vi "GF_ConfigTop16fromFile.vi"(11 "Path":path=path "N:/Configuration/Top16Config.csv") -> (2 "Top16 Array":T2(array[cluster]) {"Slope Array" format="%#.6f"; "Dig or An" format="%x"})   [LabVIEW 2016]
uses:
  <vilib>/Utility/file.llb/Read From Spreadsheet File (string).vi
panel:
  in  "Top16Cluster":T1={"Board Name"="FTSK6X4A", "Gain Array"=[0], " Slope Array"=[0.1, 0.2, 0.5, 1.0, 2.0, 5.0, 10.0, 20.0], "Offset Array"=[0.2], "Dig or An"=255, "Handle"=0, "Return"=FALSE}
  out "Rebuilt Array":string[][][](array[string])
  out "Output Array":string[][](array[string])
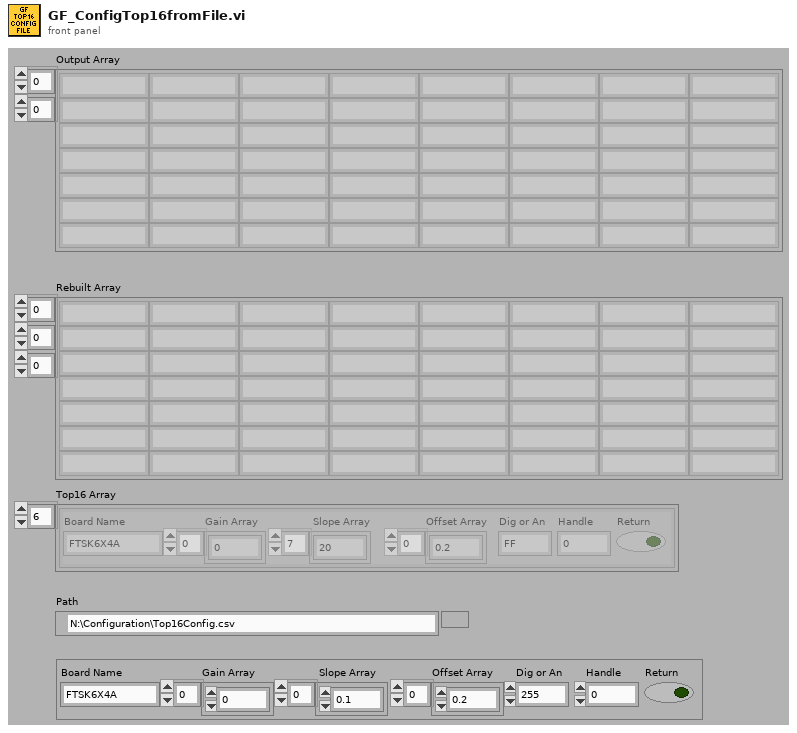
[diagram p1: front panel]
types:
  T1 = cluster{"Board Name":string, "Gain Array":u16[], " Slope Array":dbl[], "Offset Array":dbl[], "Dig or An":u8, "Handle":u32, "Return":bool}
  T2 = cluster{"Board Name":string, "Gain Array":u16[], " Slope Array":dbl[], "Offset Array":dbl[], "Dig or An":u8, "Handle":u32, "Return":bool}[]
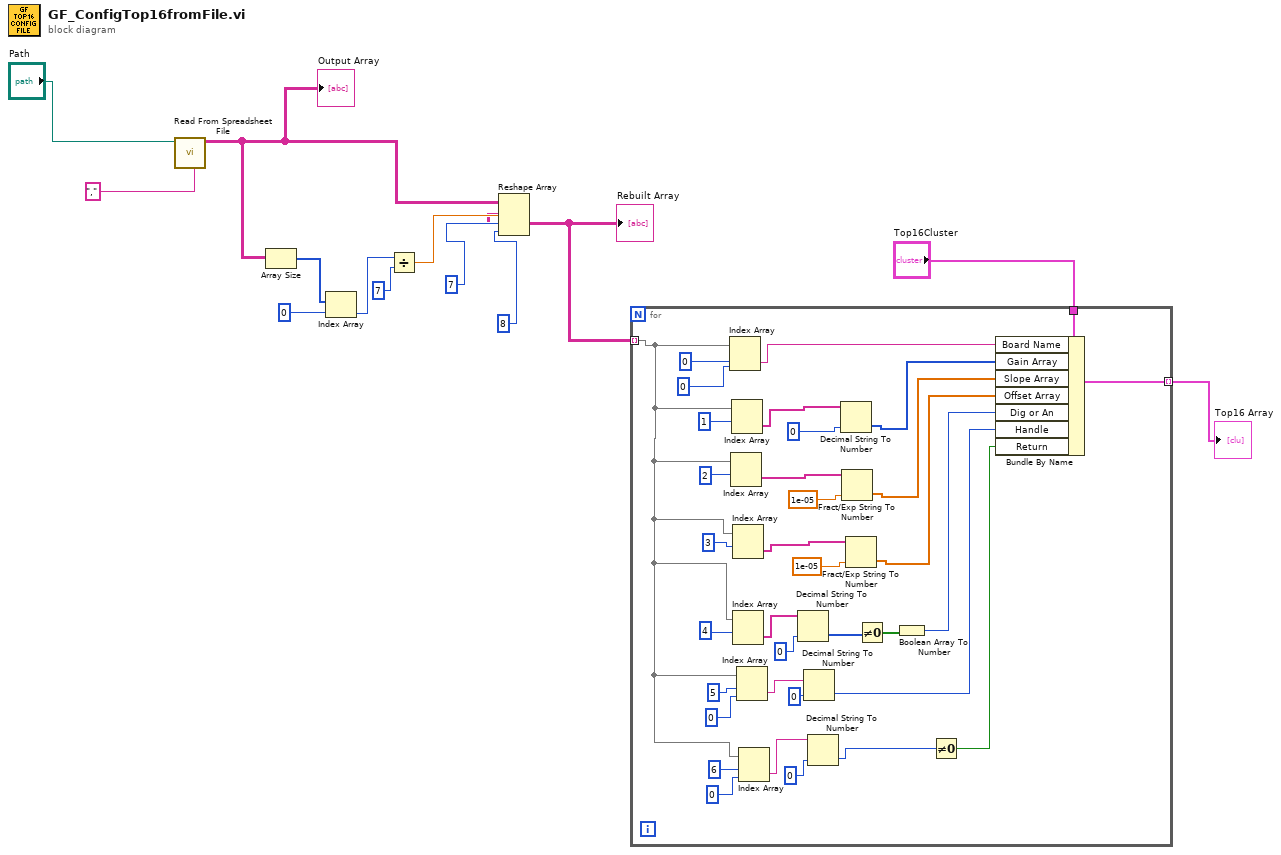
[diagram p0: block diagram]
diagram:
  n1 = call-poly <vilib>:"Read From Spreadsheet File.vi"("delimiter (\\t)"=",", "file path (dialog if empty)"="Path") -> ("all rows"=w8:string[][])  [unwired: 5 in, 4 out]
  "Output Array" <- w8
  n2 = Array Size(array=w8) -> (size(s)=w12:i32[])
  n3 = Index Array(array=w12, index=0) -> (element=w10:i32)
  n4 = Divide(x=w10, y=7) -> (x/y=w7:dbl)
  n5 = Reshape Array(w8, w7, 7, 8) -> (w4:string[][][])
  "Rebuilt Array" <- w4
  n6 = for {
    tunnel: w4 -> [w25] mode=indexing
    tunnel: [w38] -> w3 mode=indexing
    tunnel: "Top16Cluster" -> [w17]
    n7 = Index Array(array=w25, index (row)=0, index (col)=0) -> (element=w37:string)
    n8 = Index Array(array=w25, index (row)=2) -> (element=w43:string[])  [unwired: 1 in]
    n9 = Index Array(array=w25, index (row)=1) -> (element=w46:string[])  [unwired: 1 in]
    n10 = Index Array(array=w25, index (row)=3) -> (element=w40:string[])  [unwired: 1 in]
    n11 = Index Array(array=w25, index (row)=4) -> (element=w34:string[])  [unwired: 1 in]
    n12 = Index Array(array=w25, index (row)=5, index (col)=0) -> (element=w22:string)
    n13 = Index Array(array=w25, index (row)=6, index (col)=0) -> (element=w20:string)
    n14 = Decimal String To Number(string=w34, default (0L)=u8 0) -> (number=w16:u8[])  [unwired: 1 in, 1 out]
    n15 = Decimal String To Number(string=w22, default (0L)=u32 0) -> (number=w21:u32)  [unwired: 1 in, 1 out]
    n16 = Decimal String To Number(string=w20, default (0L)=u8 0) -> (number=w19:u8)  [unwired: 1 in, 1 out]
    n17 = Decimal String To Number(string=w46, default (0L)=u16 0) -> (number=w45:u16[])  [unwired: 1 in, 1 out]
    n18 = Fract/Exp String To Number(string=w43, default (0 dbl)=1e-05) -> (number=w42:dbl[])  [unwired: 2 in, 1 out]
    n19 = Fract/Exp String To Number(string=w40, default (0 dbl)=1e-05) -> (number=w39:dbl[])  [unwired: 2 in, 1 out]
    n20 = Not Equal To 0?(x=w16) -> (x != 0?=w15:bool[])
    n21 = Boolean Array To Number(Boolean array=w15) -> (number=w14:u32)
    n22 = Not Equal To 0?(x=w19) -> (x != 0?=w18:bool)
    n23 = Bundle By Name(cluster=w17, "Board Name"=w37, "Gain Array"=w45, "Slope Array"=w42, "Offset Array"=w39, "Dig or An"=w14, "Handle"=w21, "Return"=w18) -> (w38:T1)
  }
  "Top16 Array" <- w3
